vi "host_server.vi"(8 "error in (no error)":errorcluster) -> (0 "error out":errorcluster)   [LabVIEW 2021]
uses:
  host_global_vars.vi
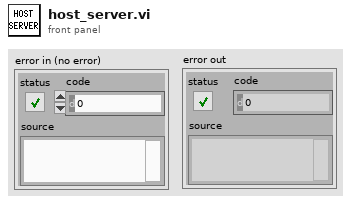
[diagram p1: front panel]
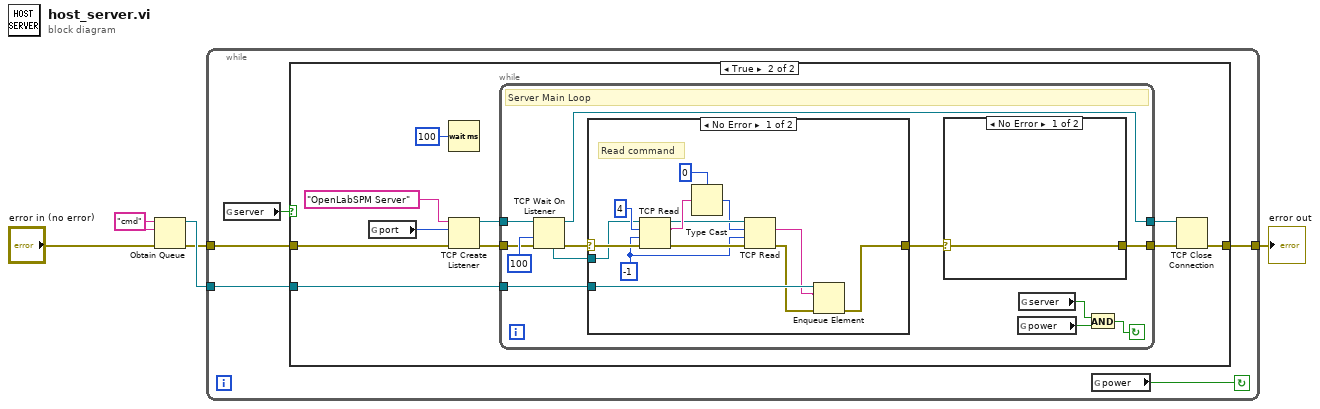
[diagram p0: block diagram]
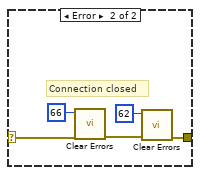
[diagram p3: hidden frame]
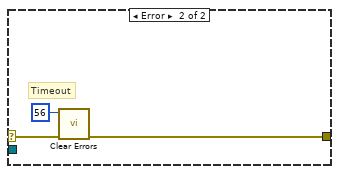
[diagram p4: hidden frame]
diagram:
  w5 = "cmd" ("name (unnamed)")
  n1 = Obtain Queue(name (unnamed)=w5, element data type=w5, error in (no error)="error in (no error)") -> (queue out=w4:refnum<queue>, error out=w3:errorcluster)  [unwired: 2 in, 1 out]
  n2 = while {
    tunnel: w4 -> [w10]
    tunnel: w3 -> [w7]
    tunnel: [w6] -> w2
    stop <- w9 continue-if-true
    n3 = global read "host_global_vars.vi" "server"() -> (w8:bool)
    n4 = case shown="True" w8 {
      tunnel: w10 -> [_ w17]
      tunnel: w7 -> [w11 w16]
      tunnel: [w11 w13] -> w6
      frame False {
      }
      frame True {
        n5 = global read "host_global_vars.vi" "port"() -> (w21:u16)
        n6 = Wait (ms)(milliseconds to wait=u32 100) -> ()  [unwired: 1 out]
        n7 = TCP Create Listener(8:w16, 10:w21, 11:"OpenLabSPM Server" ("service name")) -> (0:w18:errorcluster, 3:w19:refnum<k5>)  [unwired: 2 in, 1 out]
        n8 = while {
          tunnel: w19 -> [w32]
          tunnel: w18 -> [w31]
          tunnel: w17 -> [w29]
          tunnel: [w24] -> w14
          tunnel: [w22] -> w12
          stop <- w25 continue-if-true
          # "Server Main Loop"
          n9 = TCP Wait On Listener(8:w31, 9:100 ("timeout ms (25000)"), 11:w32) -> (0:w30:errorcluster, 3:w22:refnum<k5>, 4:w23:refnum<k5>)  [unwired: 1 in, 2 out]
          n10 = case shown="No Error" w30 {
            selector: w30 -> [w51 w54]
            tunnel: w29 -> [w44 _]
            tunnel: [w40 w53] -> w28
            tunnel: w23 -> [w42 _]
            frame No Error {
              w45 = -1 ("timeout ms (wait forever: -1)")
              # "Read command"
              n11 = TCP Read(connection ID=w42, bytes to read=4, error in (no error)=w51, 9:w45) -> (connection ID out=w48:refnum<k5>, data out=w49:string, error out=w47:errorcluster)  [unwired: 1 in]
              n12 = Type Cast(type=0 ("bytes to read"), x=w49) -> (*(type *) &x=w46:i32)
              n13 = TCP Read(connection ID=w48, bytes to read=w46, error in (no error)=w47, 9:w45) -> (data out=w43:string, error out=w41:errorcluster)  [unwired: 1 in, 1 out]
              n14 = Enqueue Element(queue=w44, element=w43, error in (no error)=w41) -> (error out=w40:errorcluster)  [unwired: 1 in, 2 out]
            }
            frame Error {
              # "Timeout"
              n15 = call <vilib>:"Clear Errors.vi"("error in (no error)"=w54, "specific error code to clear (0: all)"=56) -> ("error out"=w53:errorcluster)  [unwired: 4 in, 1 out]
            }
          }
          n16 = case shown="No Error" w28 {
            selector: w28 -> [w34 w37]
            tunnel: [w34 w35] -> w24
            frame No Error {
            }
            frame Error {
              # "Connection closed"
              n17 = call <vilib>:"Clear Errors.vi"("error in (no error)"=w37, "specific error code to clear (0: all)"=66) -> ("error out"=w36:errorcluster)  [unwired: 4 in, 1 out]
              n18 = call <vilib>:"Clear Errors.vi"("error in (no error)"=w36, "specific error code to clear (0: all)"=62) -> ("error out"=w35:errorcluster)  [unwired: 4 in, 1 out]
            }
          }
          n19 = global read "host_global_vars.vi" "power"() -> (w26:bool)
          n20 = global read "host_global_vars.vi" "server"() -> (w27:bool)
          n21 = And(x=w27, y=w26) -> (x .and. y?=w25:bool)
        }
        n22 = TCP Close Connection(connection ID=w12, error in (no error)=w14) -> (error out=w13:errorcluster)  [unwired: 1 in, 1 out]
      }
    }
    n23 = global read "host_global_vars.vi" "power"() -> (w9:bool)
  }
  "error out" <- w2
